vi "Numeric.DistributeNumber.vi"(10 "Distribution factors":dbl[](array[numeric])=[0.5, 0.3, 0.1], 11 "Number to distribute":dbl) -> (3 "Distriburion result":dbl[](array[numeric]))   [LabVIEW 2015]
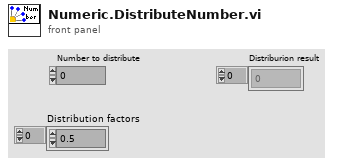
[diagram p1: front panel]
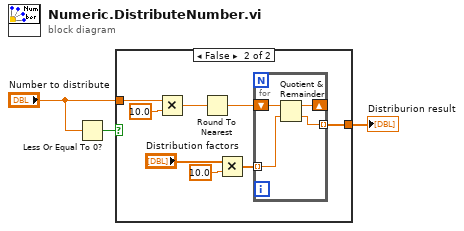
[diagram p0: block diagram]
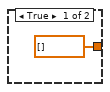
[diagram p2: hidden frame]
diagram:
  n1 = Less Or Equal To 0?(x="Number to distribute") -> (x <= 0?=w2:bool)
  n2 = case shown="False" w2 {
    tunnel: "Number to distribute" -> [_ w10]
    tunnel: [dbl[] [] w5] -> w3
    frame True {
    }
    frame False {
      n3 = Multiply(x=w10, y=10.0) -> (x*y=w11:dbl)
      n4 = Round To Nearest(number=w11) -> (nearest integer value=w9:dbl)
      n5 = Multiply(x="Distribution factors", y=10.0) -> (x*y=w6:dbl[])
      n6 = for {
        shift-right: [w15] -> _
        shift-left: w9 -> [w16]
        tunnel: w6 -> [w14] mode=indexing
        tunnel: [w13] -> w5 mode=indexing
        n7 = Quotient & Remainder(x=w16, y=w14) -> (x-y*floor(x/y)=w15:dbl, floor(x/y)=w13:dbl)
      }
    }
  }
  "Distriburion result" <- w3
